vi "Write Depth (0-1).vi"(8 "error in (no error)":errorcluster, 10 "Depth (0-1)":dbl, 11 "AM in":refnum<class "AM.lvclass">) -> (0 "error out":errorcluster, 3 "AM out":refnum<class "AM.lvclass">)   [LabVIEW 2020, in "AM.lvclass"]
uses:
  AM.lvclass
  AM.lvclass/AM.ctl
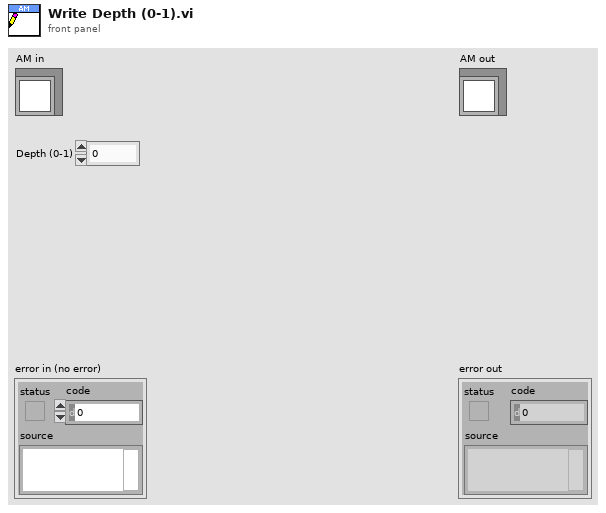
[diagram p1: front panel]
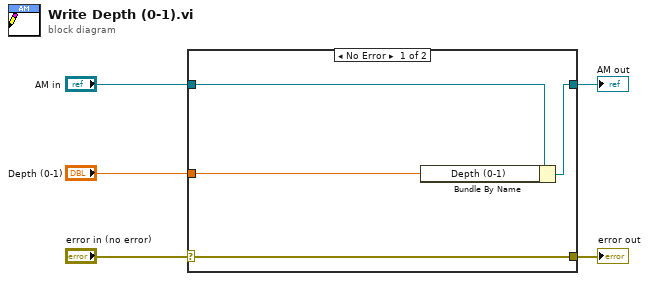
[diagram p0: block diagram]
diagram:
  n1 = case shown="No Error" "error in (no error)" {
    selector: "error in (no error)" -> [w9 w10]
    tunnel: [w9 w10] -> w4
    tunnel: [w7 w11] -> w2
    tunnel: "AM in" -> [w8 w11]
    tunnel: "Depth (0-1)" -> [w6 _]
    frame No Error {
      n2 = Bundle By Name(cluster=w8, "Depth (0-1)"=w6) -> (w7:refnum<class "AM.lvclass">)
    }
    frame Error {
    }
  }
  "error out" <- w4
  "AM out" <- w2
